vi "DAQ.Sampling.Find Integer Period Fs and Ns.vi"(10 "f integer":dbl, 11 "Max Fs":dbl) -> (3 "Timing out":T1={"Fs"=204789.0, "#s"=15753})   [LabVIEW 2019, in "Instrument.DAQ.lvclass"]
uses:
  Instrument.DAQ.lvclass
  Typedefs/DAQ.Sampling.Sampling--Cluster.ctl
panel:
  out "x":dbl
  out "Numeric":i32
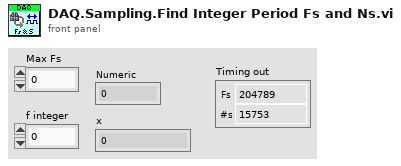
[diagram p1: front panel]
types:
  T1 = typedef "Instrument.DAQ.lvclass/DAQ.Sampling.Sampling--Cluster.ctl" = cluster{"Fs":dbl, "#s":i32}
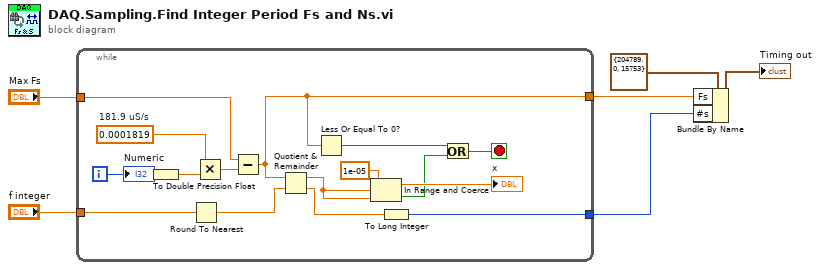
[diagram p0: block diagram]
diagram:
  n1 = while {
    tunnel: "Max Fs" -> [w20]
    tunnel: "f integer" -> [w19]
    tunnel: [w9] -> w3
    tunnel: [w8] -> w2
    i -> [w18]
    stop <- w14 stop-if-true
    w17 = 0.0001819  # 181.9 uS/s
    n2 = To Double Precision Float(number=w18) -> (double precision float=w7:dbl)
    n3 = Round To Nearest(number=w19) -> (nearest integer value=w10:dbl)
    n4 = Multiply(x=w17, y=w7) -> (x*y=w21:dbl)
    n5 = Subtract(x=w20, y=w21) -> (x-y=w8:dbl)
    n6 = Quotient & Remainder(x=w8, y=w10) -> (x-y*floor(x/y)=w15:dbl, floor(x/y)=w11:dbl)
    n7 = Less Or Equal To 0?(x=w8) -> (x <= 0?=w22:bool)
    n8 = In Range and Coerce(upper limit=1e-05, x=w15, lower limit=w15) -> (coerced(x)=→"x":dbl, In Range?=w12:bool)
    n9 = To Long Integer(number=w11) -> (32bit integer=w9:i32)
    n10 = Or(x=w22, y=w12) -> (x .or. y?=w14:bool)
    "Numeric" <- w18
  }
  n11 = Bundle By Name(cluster=T1 {"Fs"=204789.0, "#s"=15753} ("Sampling"), "Fs"=w2, "#s"=w3) -> (→"Timing out":T1)
